vi "EQ+px parameters.vi"() -> (0 "PixelReg (hex)":u32[](array[numeric]) format="%.0x", 1 "I Leak out":u8, 2 "EQ parameters (cluster) out":T1={"Timeout ITEST sweep"=21, "Number pulses ITEST"=20, "TOT"=40, "ADC target"=900, "Number pulses SSpeak sweep"=100, "Timeout SSpeak sweep"=110, "Timeout THLD sweep"=10, "Number triggers THLD sweep"=2, "First PIXEL"=0, "Last PIXEL"=99, "Sigma factor"=2, "DTP period for SSpeak sweep"=1, "Global THR for ITEST sweep"=38, "Pulse width"=0} {"Number triggers THLD sweep" step=1; "Timeout THLD sweep" step=1; "Timeout SSpeak sweep" step=1; "DTP period for SSpeak sweep" step=1; "Number pulses SSpeak sweep" step=1; "Timeout ITEST sweep" step=1; "Global THR for ITEST sweep" step=1; "Number pulses ITEST" step=1; "Pulse width" items=["25 ns", "50 ns", "75 ns", "100 ns"]; "Sigma factor" step=1; "Last PIXEL" max=99 step=1; "First PIXEL" max=99 step=1; "ADC target" step=1; "TOT" step=1})   [LabVIEW 2015, in "VIPM2.lvlib"]
doc: "New window to set EQ and pixel configuration."
uses:
  VIPM2.lvlib
panel:
  in  "Default Button":bool
  in  "Execute Button":bool
  in  "I feed range":bool
  in  "SS gain":fxp<+,2,2>=3.0
  in  "PA gain":fxp<+,2,2>
  in  "I Leak":fxp<+,2,2>=1.0
  in  "EQ parameters (cluster)":T2={"Number pulses ITEST"=20, "TOT"=40, "ADC target"=900, "Number triggers THLD sweep"=2, "ACQ GbTHLD"=38, "Pulse width"=0} caption="EQ parameters" {"Pulse width" items=["25 ns", "50 ns", "75 ns", "100 ns"]; "ACQ GbTHLD" items=["0.34", "0.37", "0.40", "0.43", "0.45", "0.48", "0.51", "0.54", "0.57", "0.60", "0.63", "0.65", "0.68", "0.71", "0.74", "0.77", "0.80", "0.82", "0.85", "0.88", "0.91", "0.94", "0.97", "0.99", "1.02", "1.05", "1.08", "1.11", "1.14", "1.16", "1.19", "1.22", "1.25", "1.28", "1.31", "1.34", "1.36", "1.39", "1.42", "1.45", "1.48", "1.51", "1.53", "1.56", "1.59", "1.62", "1.65", "1.68", "1.70", "1.73", "1.76", "1.79", "1.82", "1.85", "1.88", "1.90", "1.93", "1.96", "1.99", "2.02", "2.05", "2.07", "2.10", "2.13"]; "Number triggers THLD sweep" step=1; "Number pulses ITEST" step=1; "ADC target" step=1; "TOT" step=1}
  # "Set parameters"
  # "Pixel parameters"
  # "I test sweep"
  # "SS peak sweep"
  # "THLD sweep"
  # "Number of triggers"
  # "Timeout"
  # "Timeout"
  # "DTP period"
  # "Number of pulses"
  # "Timeout"
  # "Global THR"
  # "Number of pulses"
  # "I test sweep"
  # "SS peak sweep"
  # "THLD sweep"
  # "Number of triggers"
  # "Number of pulses"
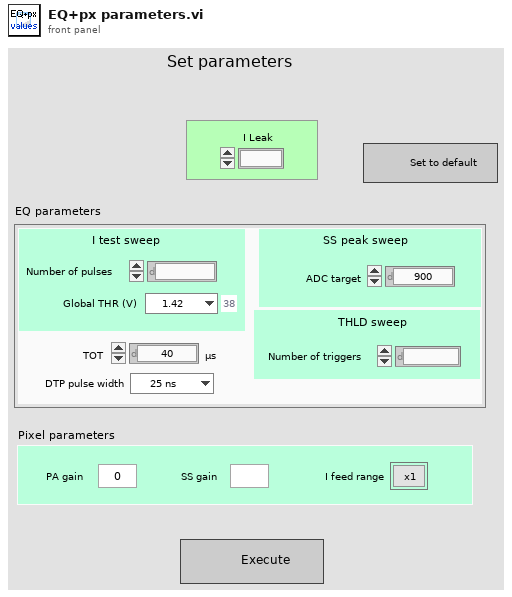
[diagram p1: front panel]
types:
  T1 = cluster{"Timeout ITEST sweep":u32, "Number pulses ITEST":u32, "TOT":u32, "ADC target":u32, "Number pulses SSpeak sweep":u32, "Timeout SSpeak sweep":u32, "Timeout THLD sweep":u32, "Number triggers THLD sweep":u32, "First PIXEL":u32, "Last PIXEL":u32, "Sigma factor":u32, "DTP period for SSpeak sweep":u32, "Global THR for ITEST sweep":u32, "Pulse width":u32}
  T2 = cluster{"Number pulses ITEST":u32, "TOT":u32, "ADC target":u32, "Number triggers THLD sweep":u32, "ACQ GbTHLD":u8, "Pulse width":u32}
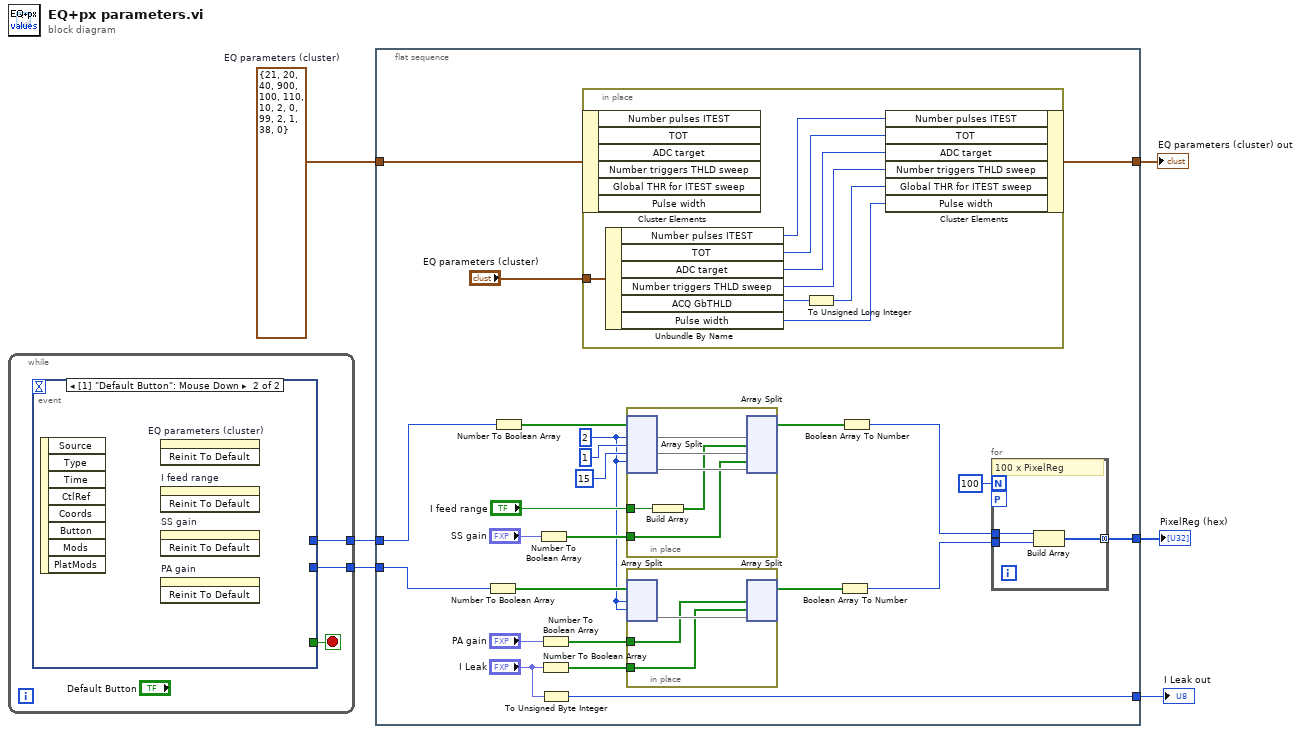
[diagram p0: block diagram]
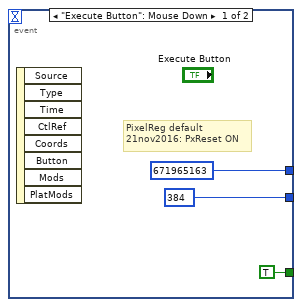
[diagram p2: hidden frame]
diagram:
  w3 = T1 {"Timeout ITEST sweep"=21, "Number pulses ITEST"=20, "TOT"=40, "ADC target"=900, "Number pulses SSpeak sweep"=100, "Timeout SSpeak sweep"=110, "Timeout THLD sweep"=10, "Number triggers THLD sweep"=2, "First PIXEL"=0, "Last PIXEL"=99, "Sigma factor"=2, "DTP period for SSpeak sweep"=1, "Global THR for ITEST sweep"=38, "Pulse width"=0}  # EQ parameters (cluster)
  n1 = while {
    tunnel: [w9] -> w6
    tunnel: [w8] -> w5
    stop <- w7 stop-if-true
    n2 = event shown="[1] \"Default Button\": Mouse Down" {
      selector: _ -> [_ _]
      dyn-events: _ -> [_ _]
      timeout: _ -> [_ _]
      tunnel: [u32 671965163 ("Numeric") _] -> w9
      tunnel: [u32 384 ("x") _] -> w8
      tunnel: [TRUE _] -> w7
      event "Execute Button": Mouse Down {
        # "PixelReg default\n21nov2016: PxReset ON"
        n3 = event-data() -> ()  [unwired: 1 in, 8 out]
      }
      event "Default Button": Mouse Down {
        n4 = event-data() -> ()  [unwired: 1 in, 8 out]
        n5 = invoke on="EQ parameters (cluster)" class="Clust (strict)" method="Reinit To Default"() -> ()  [unwired: 3 in, 3 out]
        n6 = invoke on="I feed range" class="Bool (strict)" method="Reinit To Default"() -> ()  [unwired: 3 in, 3 out]
        n7 = invoke on="SS gain" class="DigNum (strict)" method="Reinit To Default"() -> ()  [unwired: 3 in, 3 out]
        n8 = invoke on="PA gain" class="DigNum (strict)" method="Reinit To Default"() -> ()  [unwired: 3 in, 3 out]
      }
    }
  }
  n9 = flat-sequence {
    tunnel: w6 -> [w36]
    tunnel: w5 -> [w28]
    tunnel: [w18] -> w4
    tunnel: w3 -> [w17]
    tunnel: [w16] -> w2
    tunnel: [w13] -> w1
    frame #0 {
      w26 = 2
      n10 = Number To Boolean Array(number=w28) -> (Boolean array=w27:bool[])
      n11 = Number To Boolean Array(number=w36) -> (Boolean array=w33:bool[])
      n12 = Number To Boolean Array(number="SS gain") -> (Boolean array=w29:bool[])
      n13 = Number To Boolean Array(number="PA gain") -> (Boolean array=w25:bool[])
      n14 = Number To Boolean Array(number="I Leak") -> (Boolean array=w24:bool[])
      n15 = To Unsigned Byte Integer(number="I Leak") -> (unsigned 8bit integer=w13:u8)
      n16 = in-place {
        in-place-border: "EQ parameters (cluster)" -> [w44]
        n17 = in-place-cluster #1(w17) -> ()  [unwired: 6 out]
        n18 = Unbundle By Name(w44) -> ("Number pulses ITEST"=w43:u32, "TOT"=w42:u32, "ADC target"=w41:u32, "Number triggers THLD sweep"=w40:u32, "ACQ GbTHLD"=w39:u8, "Pulse width"=w37:u32)
        n19 = To Unsigned Long Integer(number=w39) -> (unsigned 32bit integer=w38:u32)
        n20 = in-place-cluster #1("Number pulses ITEST"=w43, "TOT"=w42, "ADC target"=w41, "Number triggers THLD sweep"=w40, "Global THR for ITEST sweep"=w38, "Pulse width"=w37) -> (w16:T1)
      }
      n21 = in-place {
        in-place-border: "I feed range" -> [w53]
        in-place-border: w29 -> [w51]
        n22 = in-place-split #2(w33, w26, 1, 15, w26) -> (w56:bool[], w55:bool[], w54:bool[])  [unwired: 2 out]
        n23 = Build Array(w53) -> (w52:bool[])
        n24 = in-place-split #2(w56, w52, w55, w51, w54) -> (w23:bool[])  [unwired: 4 out]
      }
      n25 = in-place {
        in-place-border: w25 -> [w49]
        in-place-border: w24 -> [w48]
        n26 = in-place-split #3(w27, w26, w26) -> (w50:bool[])  [unwired: 2 out]
        n27 = in-place-split #3(w49, w48, w50) -> (w22:bool[])  [unwired: 2 out]
      }
      n28 = Boolean Array To Number(Boolean array=w22) -> (number=w19:u32)
      n29 = Boolean Array To Number(Boolean array=w23) -> (number=w20:u32)
      n30 = for {
        N: 100 -> [_]
        tunnel: w20 -> [w47]
        tunnel: w19 -> [w46]
        tunnel: [w45] -> w18 mode=concatenating
        workers-P: _ -> [_]
        # "100 x PixelReg"
        n31 = Build Array "Build Array"(w47, w46) -> (w45:u32[])
      }
    }
  }
  "PixelReg (hex)" <- w4
  "EQ parameters (cluster) out" <- w2
  "I Leak out" <- w1
